vi "13_EventLogger.vi"(8 "error in (no error)":errorcluster) -> (0 "error out":errorcluster)   [LabVIEW 2014]
uses:
  SwabianInstruments.TimeTagger
panel:
  out "Events log":string
  in  "stop":bool
  # "This example shows how to capture the .NET events in LabView.\nThe TimeTagger software uses Events to send information and error messages to the client programs.\nThe exceptions in the method calls are sent to the LabVIEW error line as usual.\n\nRun the VI.\n\nUnplug the USB cable from the Time Tagger.\n\nWhen you unplug the cable the Time Tagger software will report connection problem that will be displayed in the text field below."
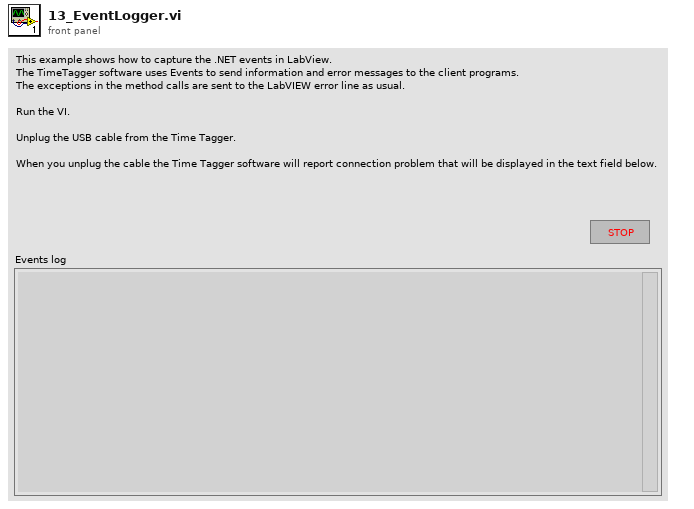
[diagram p1: front panel]
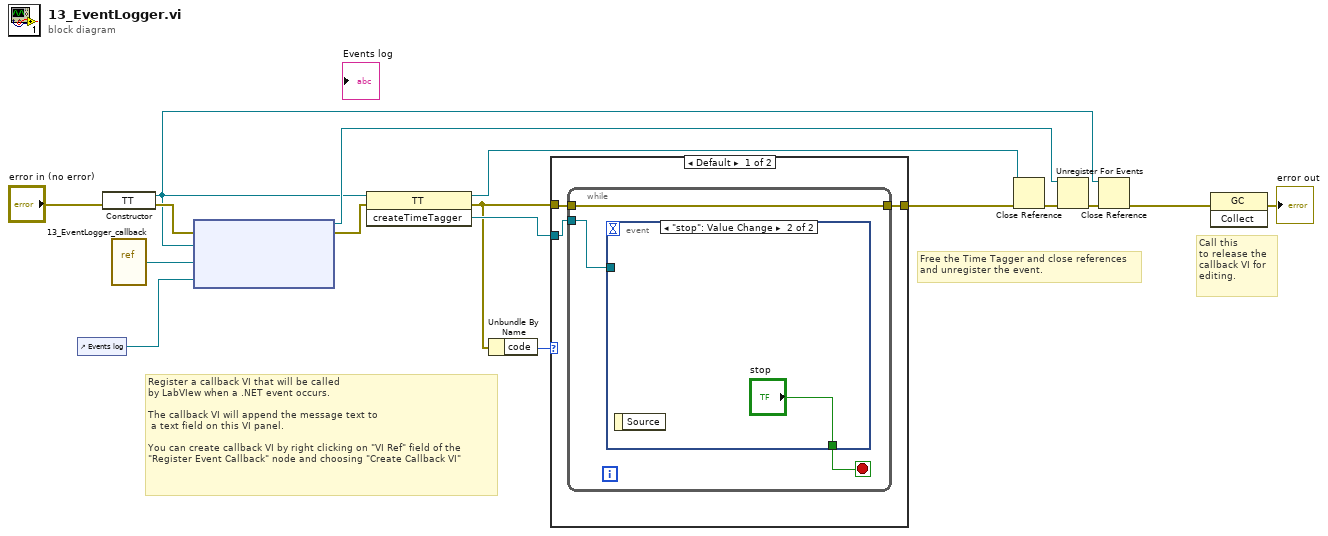
[diagram p0: block diagram]
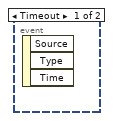
[diagram p2: hidden frame]
diagram:
  # "Free the Time Tagger and close references\nand unregister the event."
  # "Register a callback VI that will be called \nby LabVIew when a .NET event occurs.\n\nThe callback VI will append the message text to\n a text field on this VI panel.\n\nYou can create callback VI by right clicking on \"VI Ref\" field of the \n\"Register Event Callback\" node and choosing \"Create Callback VI\""
  # "Call this \nto release the \ncallback VI for \nediting."
  n1 = control-ref of="Events log"() -> (w15:refnum<vi>)
  n2 = constructor class="TT"(error in="error in (no error)") -> (reference out=w1:refnum<k24>, error out=w10:errorcluster)  [unwired: 2 in, 1 out]
  n3 = vi-ref "13_EventLogger_callback.vi"() -> ("vi reference"=w8:refnum<vi>)
  n4 = node(w10, w1, w8, w15) -> (w16:refnum<k27>, w9:errorcluster)  [unwired: 1 in]
  n5 = invoke class="TT" method="createTimeTagger"(reference=w1, error in=w9) -> (reference out=w6:refnum<k24>, error out=w3:errorcluster, "createTimeTagger"=w13:refnum<k24>)  [unwired: 1 in]
  n6 = Unbundle By Name(w3) -> ("code"=w2:i32)
  n7 = case shown="Default" w2 {
    tunnel: w13 -> [w19 _]
    tunnel: w3 -> [w18 w24]
    tunnel: [w17 w24] -> w7
    frame Default {
      n8 = while {
        tunnel: w18 -> [w20]
        tunnel: [w20] -> w17
        tunnel: w19 -> [w21]
        stop <- w22 stop-if-true
        n9 = event shown="[1] \"stop\": Value Change" {
          selector: _ -> [_ _]
          dyn-events: _ -> [_ _]
          timeout: _ -> [_ _]
          tunnel: [_ "stop"] -> w22
          tunnel: w21 -> [_ _]
          event Timeout {
            n10 = event-data() -> ()  [unwired: 1 in, 3 out]
          }
          event "stop": Value Change {
            n11 = event-data() -> ()  [unwired: 1 in, 1 out]
          }
        }
      }
    }
    frame 43981 {
      # "This case allows to avoid\nwaiting for user input. It\nis just important for automated\ntesting - you can ignore it."
    }
  }
  n12 = Close Reference(reference=w6, error in (no error)=w7) -> (error out=w12:errorcluster)
  n13 = Unregister For Events(event registration refnum=w16, error in=w12) -> (error out=w14:errorcluster)
  n14 = Close Reference(reference=w1, error in (no error)=w14) -> (error out=w11:errorcluster)
  n15 = invoke class="GC" method="Collect"(error in=w11) -> (error out=→"error out":errorcluster)  [unwired: 2 in, 2 out]
